vi "Stereo - Get Max Pixel Value.vi"(8 "error in (no error)":errorcluster, 11 "Image":T1) -> (0 "error out":errorcluster, 1 "Color Palette":cluster{"Red":u8, "Green":u8, "Blue":u8}[](array[cluster]), 2 "Max Value":dbl, 3 "Image dup":T1)   [LabVIEW 2017]
doc: "Returns the max pixel value of a grayscale image, and builds a color palette with the max value being red."
uses:
  <vilib>/vision/Image Controls.llb/IMAQ Image.ctl
panel:
  # "Overview: Returns the max pixel value of a grayscale image, and builds a color palette with the max value being red."
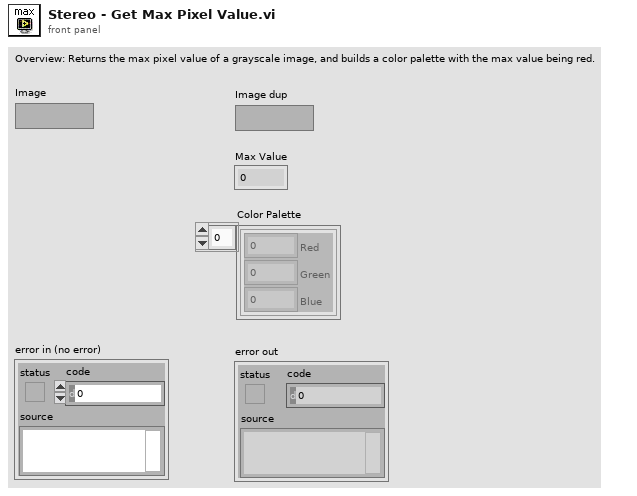
[diagram p1: front panel]
types:
  T1 = typedef "IMAQ Image.ctl" = refnum<image>
  T2 = typedef "Image Type" = u32
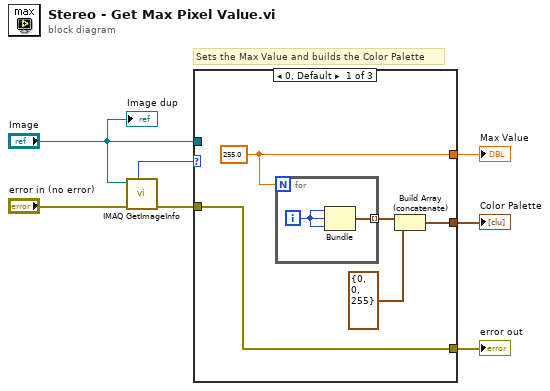
[diagram p0: block diagram]
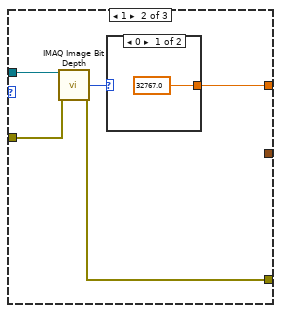
[diagram p2: hidden frame]
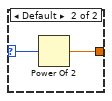
[diagram p3: hidden frame]
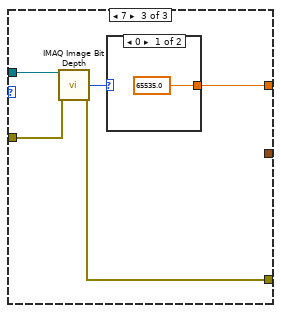
[diagram p4: hidden frame]
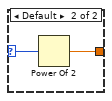
[diagram p5: hidden frame]
diagram:
  # "Sets the Max Value and builds the Color Palette"
  n1 = call "IMAQ GetImageInfo"("error in (no error)"="error in (no error)", "Image"="Image") -> ("error out"=w2:errorcluster, "Image Type"=w7:T2)  [unwired: 8 out]
  n2 = case shown="0, Default" w7 {
    tunnel: [w12 w19 w27] -> w6
    tunnel: [w10 _ _] -> w5
    tunnel: "Image" -> [_ w17 w25]
    tunnel: w2 -> [w8 w16 w24]
    tunnel: [w8 w15 w23] -> w1
    frame 0, Default {
      w12 = 255.0
      n3 = for {
        N: w12 -> [_]
        tunnel: [w13] -> w11 mode=indexing
        i -> [w14]
        n4 = Bundle(w14, w14, w14) -> (w13:cluster{i32, i32, i32})  [unwired: 1 out]
      }
      n5 = Build Array (concatenate)(w11, cluster{"Red":u8, "Green":u8, "Blue":u8} {"Red"=0, "Green"=0, "Blue"=255}) -> (w10:cluster{"Red":i32, "Green":i32, "Blue":i32}[])
    }
    frame 1 {
      n6 = call "IMAQ Image Bit Depth"("Image"=w17, "error in (no error)"=w16) -> ("Bit Depth"=w18:u32, "error out"=w15:errorcluster)  [unwired: 2 in, 10 out]
      n7 = case shown="0" w18 {
        selector: w18 -> [_ w21]
        tunnel: [32767.0 w22] -> w19
        frame 0 {
        }
        frame Default {
          n8 = Power Of 2(x=w21) -> (2^x=w22:dbl)
        }
      }
    }
    frame 7 {
      n9 = call "IMAQ Image Bit Depth"("Image"=w25, "error in (no error)"=w24) -> ("Bit Depth"=w26:u32, "error out"=w23:errorcluster)  [unwired: 2 in, 10 out]
      n10 = case shown="0" w26 {
        selector: w26 -> [_ w29]
        tunnel: [65535.0 w30] -> w27
        frame 0 {
        }
        frame Default {
          n11 = Power Of 2(x=w29) -> (2^x=w30:dbl)
        }
      }
    }
  }
  "Max Value" <- w6
  "Color Palette" <- w5
  "error out" <- w1
  "Image dup" <- "Image"
